vi "Close.vi"(8 "error in (no error)":errorcluster caption="entrée d'erreur (pas d'erreur)", 11 "Class Relay_Board 16_Relay_R4D3D16 en entrée":refnum<class "Class Relay_Board 8_Relay_N4D8B08.lvclass">) -> (0 "error out":errorcluster caption="sortie d'erreur", 3 "Class Relay_Board 16_Relay_R4D3D16 en sortie":refnum<class "Class Relay_Board 8_Relay_N4D8B08.lvclass">)   [LabVIEW 2020, in "Library Instrument & Equipement.lvlib" / "Library Relay_Board.lvlib" / "Class Relay_Board 8_Relay_N4D8B08.lvclass"]
uses:
  Class Relay_Board 8_Relay_N4D8B08.lvclass
  C:/Users/ngarcin/OneDrive - Altyor/Standard TB/Class/Relay_Board/Relay_Board (Default)/Class Relay_Board (Default).lvclass
  Modbus/Modbus.lvclass
  Class Relay_Board 8_Relay_N4D8B08.lvclass/Class Relay_Board 8_Relay_N4D8B08.ctl
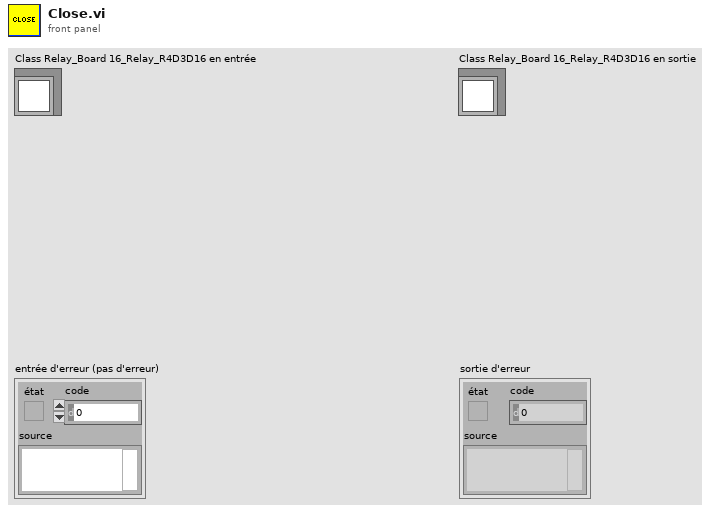
[diagram p1: front panel]
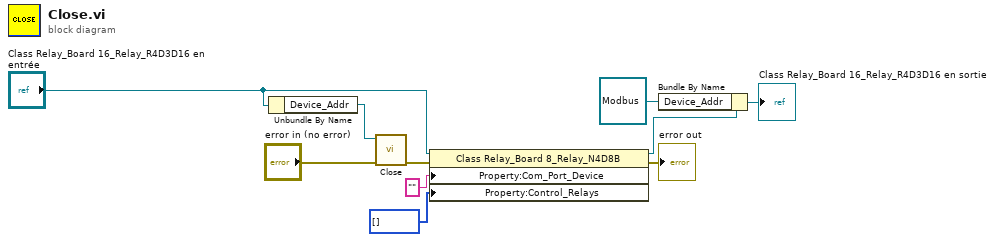
[diagram p0: block diagram]
diagram:
  n1 = Unbundle By Name("Class Relay_Board 16_Relay_R4D3D16 en entrée") -> ("Device_Addr"=w2:refnum<class "Modbus.lvclass">)
  n2 = call-dynamic "Close.vi"("error in (no error)"="error in (no error)", "MODBUS in"=w2) -> ("error out"=w3:errorcluster)  [unwired: 9 in]
  n3 = property class="Class Relay_Board 8_Relay_N4D8B"(reference="Class Relay_Board 16_Relay_R4D3D16 en entrée", error in=w3, "Property:Com_Port_Device"="" ("Address_Device"), "Property:Control_Relays"=u8[] [] ("Control_Relays")) -> (reference out=w6:refnum<class "Class Relay_Board 8_Relay_N4D8B08.lvclass">, error out=→"error out":errorcluster)
  n4 = Bundle By Name(cluster=w6, "Device_Addr"=refnum<class "Modbus.lvclass"> refnum) -> (→"Class Relay_Board 16_Relay_R4D3D16 en sortie":refnum<class "Class Relay_Board 8_Relay_N4D8B08.lvclass">)
